vi "InitConnection.vi"(8 "ErrorIn":errorcluster, 11 "IsRealRobot":bool) -> (0 "ErrorOut":errorcluster, 3 "Connection":T1)   [LabVIEW 2019]
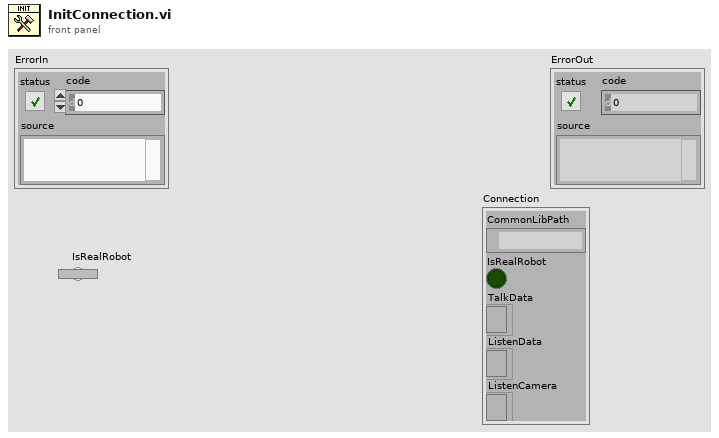
[diagram p1: front panel]
types:
  T1 = cluster{"CommonLibPath":path, "IsRealRobot":bool, "TalkData":refnum<k5>, "ListenData":refnum<k5>, "ListenCamera":refnum<k5>}
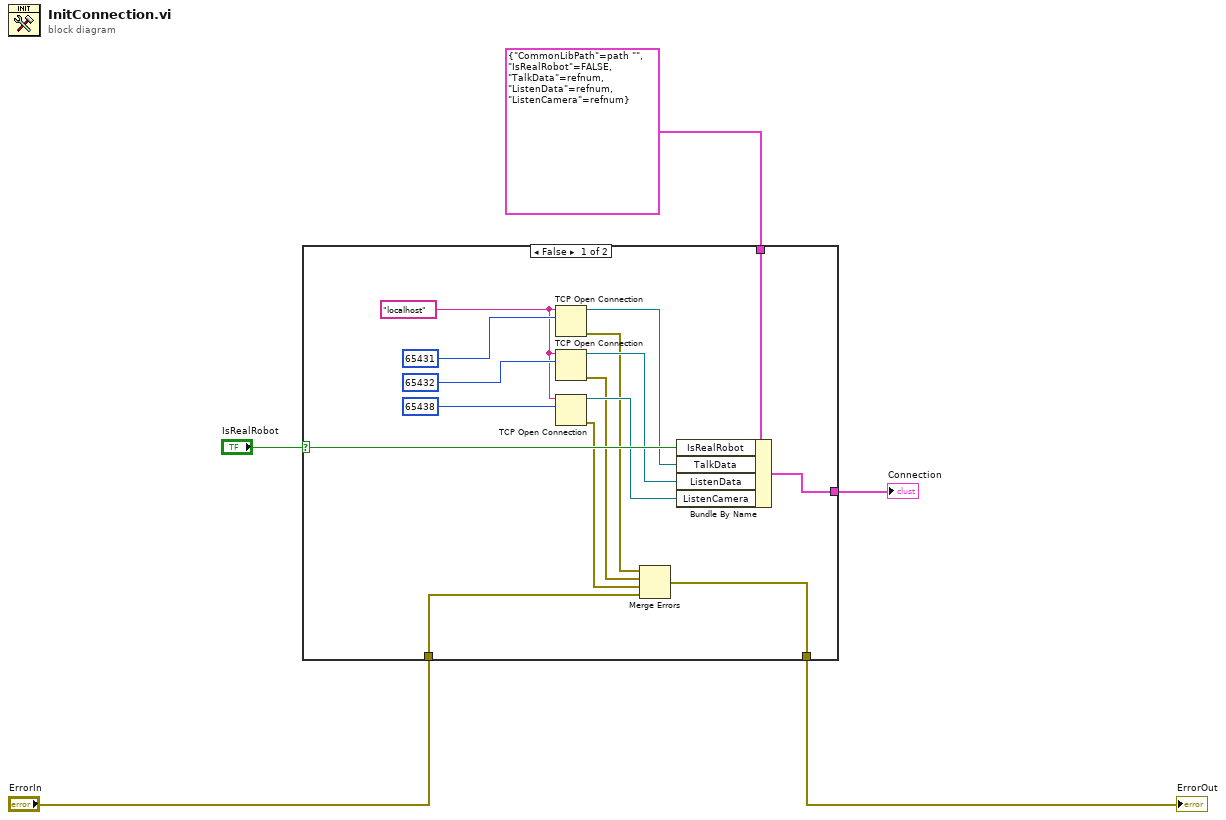
[diagram p0: block diagram]
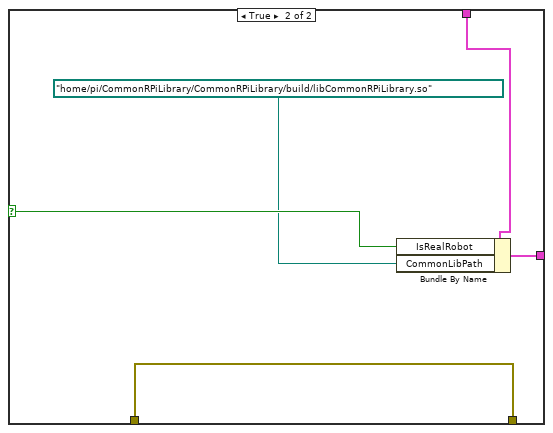
[diagram p2: hidden frame]
diagram:
  n1 = case shown="False" "IsRealRobot" {
    selector: "IsRealRobot" -> [w18 w23]
    tunnel: [w10 w21] -> w5
    tunnel: [w20 w25] -> w1
    tunnel: "ErrorIn" -> [w11 w21]
    tunnel: T1 {"CommonLibPath"=path "", "IsRealRobot"=FALSE, "TalkData"=refnum, "ListenData"=refnum, "ListenCamera"=refnum} -> [w19 w24]
    frame False {
      w6 = "localhost" ("address")
      n2 = TCP Open Connection(address=w6, remote port or service name=u16 65431 ("port")) -> (connection ID=w14:refnum<k5>, error out=w9:errorcluster)  [unwired: 3 in]
      n3 = TCP Open Connection(address=w6, remote port or service name=u16 65432 ("port")) -> (connection ID=w13:refnum<k5>, error out=w8:errorcluster)  [unwired: 3 in]
      n4 = TCP Open Connection(address=w6, remote port or service name=u16 65438 ("port")) -> (connection ID=w12:refnum<k5>, error out=w7:errorcluster)  [unwired: 3 in]
      n5 = Merge Errors(w9, w8, w7, w11) -> (w10:errorcluster)
      n6 = Bundle By Name(cluster=w19, "IsRealRobot"=w18, "TalkData"=w14, "ListenData"=w13, "ListenCamera"=w12) -> (w20:T1)
    }
    frame True {
      n7 = Bundle By Name(cluster=w24, "IsRealRobot"=w23, "CommonLibPath"=path "/home/pi/CommonRPiLibrary/CommonRPiLibrary/build/libCommonRPiLibrary.so" ("path in")) -> (w25:T1)
    }
  }
  "ErrorOut" <- w5
  "Connection" <- w1
